vi "Set Speed.vi"(8 "error in (no error)":errorcluster, 10 "Speed":enum16{"Slow Speed", "High Speed"}(ring), 11 "FW102C in":i32) -> (0 "error out":errorcluster, 3 "FW102C out":i32)   [LabVIEW 2015, in "Thorlabs_FW102C.lvlib"]
doc: "speed=0 Sets the move profile to slow speed\nspeed=1 Sets the move profile to high speed"
uses:
  Thorlabs_FW102C.lvlib
  Library/FilterWheel102_win32.dll
  <instrlib>/Thorlabs_FW102C/Library/FilterWheel102_win64.dll
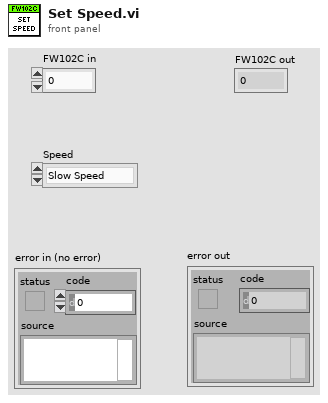
[diagram p1: front panel]
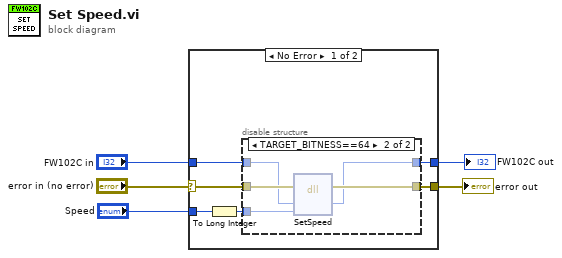
[diagram p0: block diagram]
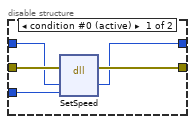
[diagram p2: hidden frame]
diagram:
  n1 = case shown="No Error" "error in (no error)" {
    selector: "error in (no error)" -> [w11 w22]
    tunnel: [w10 w22] -> w5
    tunnel: "FW102C in" -> [w9 w23]
    tunnel: [w8 w23] -> w2
    tunnel: "Speed" -> [w7 _]
    frame No Error {
      n2 = To Long Integer(number=w7) -> (32bit integer=w6:i32)
      n3 = disable-structure shown="TARGET_BITNESS==64" {
        disable-tunnel: w11 -> [w16 w21]
        disable-tunnel: [w15 w20] -> w10
        disable-tunnel: w9 -> [w14 w19]
        disable-tunnel: [w13 w18] -> w8
        disable-tunnel: w6 -> [w12 w17]
        frame condition #0 (active) {
          n4 = dll-call lib="C:/Users/bspok/Desktop/AppNotes_FW102C_v400/AppNotes_FW102C/LabVIEW/Thorlabs_FW102C/Library/FilterWheel102_win32.dll" fn="SetSpeed"(error in=w16, "hdl"=w14, "speed"=w12) -> (error out=w15:errorcluster, "hdl"=w13:i32)  [unwired: 4 in, 1 out]
        }
        frame condition #1 {
          n5 = dll-call lib="D:/Program Files/National Instruments/LabVIEW 2011/instr.lib/Thorlabs_FW102C/Library/FilterWheel102_win64.dll" fn="SetSpeed"(error in=w21, "hdl"=w19, "speed"=w17) -> (error out=w20:errorcluster, "hdl"=w18:i32)  [unwired: 4 in, 1 out]
        }
      }
    }
    frame Error {
    }
  }
  "error out" <- w5
  "FW102C out" <- w2
